vi "While.vi"() -> ()   [LabVIEW 2020]
panel:
  out "Numeric 4":i32
  in  "BREAK":bool
  out "Numeric 3":dbl
  in  "Numeric 2":dbl
  in  "Numeric":dbl
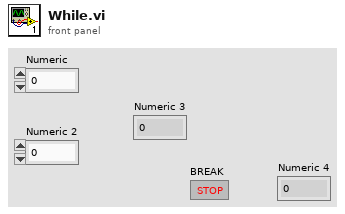
[diagram p1: front panel]
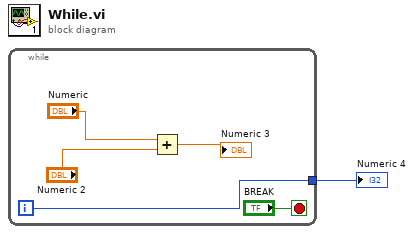
[diagram p0: block diagram]
diagram:
  n1 = while {
    tunnel: [w2] -> w1
    i -> [w2]
    stop <- "BREAK" stop-if-true
    n2 = Add(x="Numeric", y="Numeric 2") -> (x+y=→"Numeric 3":dbl)
  }
  "Numeric 4" <- w1
